vi "set_roi_color.vi"(6 "enable ROI numbering":bool caption="enable numbering", 8 "error in (no error)":errorcluster, 10 "ROI color":u32(colorbox)=15859456, 11 "TrajectoryMH100122AODRAPS in":refnum<class "TrajectoryMH100122AODRAPS.lvclass">) -> (0 "error out":errorcluster, 3 "TrajectoryMH100122AODRAPS out":refnum<class "TrajectoryMH100122AODRAPS.lvclass">)   [LabVIEW 2010, in "TrajectoryMH100122AODRAPS.lvclass"]
uses:
  TrajectoryMH100122AODRAPS.lvclass
  TrajectoryMH100122AODRAPS.lvclass/TrajectoryMH100122AODRAPS.ctl
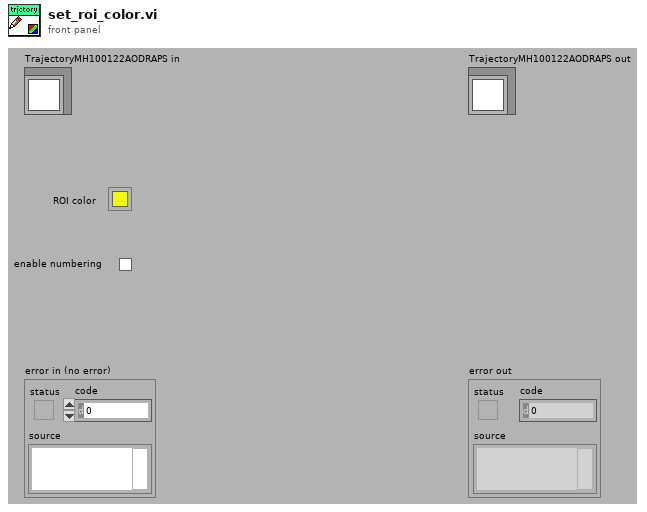
[diagram p1: front panel]
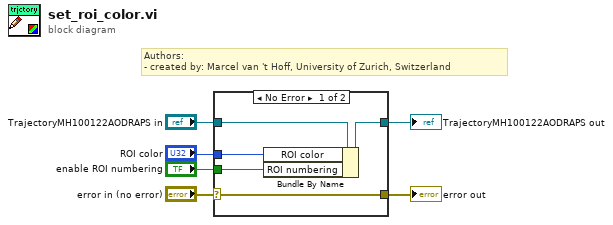
[diagram p0: block diagram]
diagram:
  # "Authors: \n- created by: Marcel van 't Hoff, University of Zurich, Switzerland"
  n1 = case shown="No Error" "error in (no error)" {
    selector: "error in (no error)" -> [w11 w13]
    tunnel: [w11 w13] -> w5
    tunnel: [w9 w12] -> w3
    tunnel: "TrajectoryMH100122AODRAPS in" -> [w10 w12]
    tunnel: "ROI color" -> [w8 _]
    tunnel: "enable ROI numbering" -> [w7 _]
    frame No Error {
      n2 = Bundle By Name(cluster=w10, "ROI color"=w8, "ROI numbering"=w7) -> (w9:refnum<class "TrajectoryMH100122AODRAPS.lvclass">)
    }
    frame Error {
    }
  }
  "error out" <- w5
  "TrajectoryMH100122AODRAPS out" <- w3
